vi "SetSlitwidth.vi"(8 "error in (no error)":errorcluster, 9 "Slitwidth":u16, 10 "Slit":T1(ring), 11 "HRS_Spectrometer in":refnum<class "HRS_Spectrometer.lvclass">) -> (0 "error out":errorcluster, 3 "HRS_Spectrometer out":refnum<class "HRS_Spectrometer.lvclass">)   [LabVIEW 2023, in "HRS_Spectrometer.lvlib" / "HRS_Spectrometer.lvclass"]
uses:
  HRS_Spectrometer.lvclass
  HRS_Spectrometer.lvclass/HRS_Spectrometer.ctl
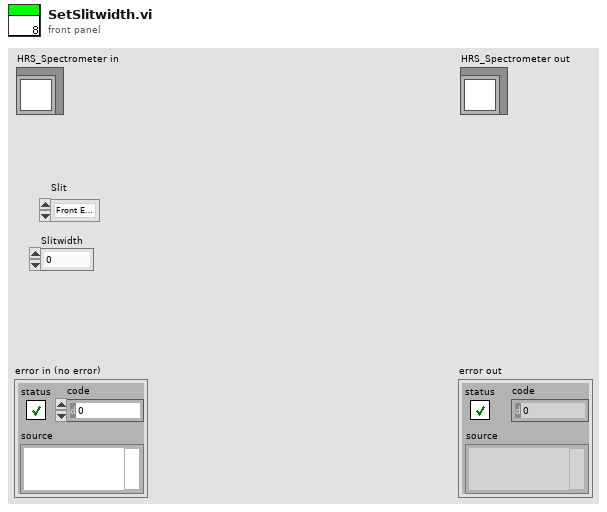
[diagram p1: front panel]
types:
  T1 = enum16{"Front Entrance Slit", "Side Entrance Slit", "Front Exit Slit", "Side Exit Slit"}
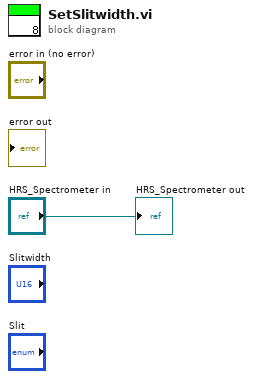
[diagram p0: block diagram]
diagram:
  "HRS_Spectrometer out" <- "HRS_Spectrometer in"
